vi "PH_Beamline.set Switch GUI in GUI.vi"(0 "i ref in":refnum<vi>, 1 "Boolean GUI Ref":refnum<vi>, 3 "Status":T1 items=["no info", "off/false/out", "on/true/in", "Failure", "Alarm", "Status 1", "Status 2", "Status 3"], 5 "error in":errorcluster) -> (14 "i ref out":refnum<vi>, 19 "error out":errorcluster)   [LabVIEW 2014, in "PH_Beamline.lvlib"]
doc: "This VI sets the Switch GUI State GUI object."
uses:
  PH_Beamline.lvlib
  PH_Basics/PH_StatusHandler/PH_StatusHandler.Status.ctl
  PH_Basics/PH_Common/PH_Common.lvlib
  PH_Basics/PH_StatusHandler/PH_StatusHandler.lvlib
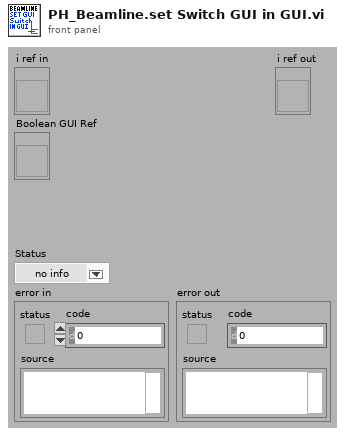
[diagram p1: front panel]
types:
  T1 = typedef "PH_StatusHandler.lvlib/PH_StatusHandler.Status.ctl" = i16
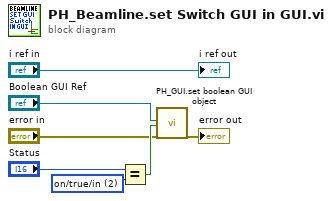
[diagram p0: block diagram]
diagram:
  w5 = T1 2 items=["no info", "off/false/out", "on/true/in", "Failure", "Alarm", "Status 1", "Status 2", "Status 3"] ("Status 2")
  n1 = Equal?(x="Status", y=w5) -> (x = y?=w4:bool)
  n2 = call "PH_GUI.set boolean GUI object.vi"("Boolean Knob GUI Ref"="Boolean GUI Ref", "Value"=w4, "error in (no error)"="error in") -> ("error out"=→"error out":errorcluster)  [unwired: 16 in]
  "i ref out" <- "i ref in"
